vi "Create Unique Child Item Name.vi"(8 "error in (no error)":errorcluster, 10 "Name in":string, 11 "Parent Item Ref in":T1=18446744073709551615 format="%.0x") -> (0 "error out":errorcluster, 2 "Unique Name out":string, 3 "Parent Item Ref out":T1=18446744073709551615 format="%.0x")   [LabVIEW 2015, in "Waveform Data Logger System Explorer.lvlib"]
uses:
  Waveform Data Logger System Explorer.lvlib
  <vilib>/NI Veristand/Custom Device API/Custom Device Item Ref.ctl
  <vilib>/NI VeriStand/Custom Device API/Custom Device API.lvlib
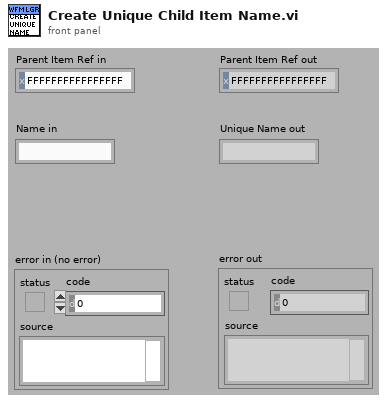
[diagram p1: front panel]
types:
  T1 = typedef "Custom Device API.lvlib/Custom Device Item Ref.ctl" = u64
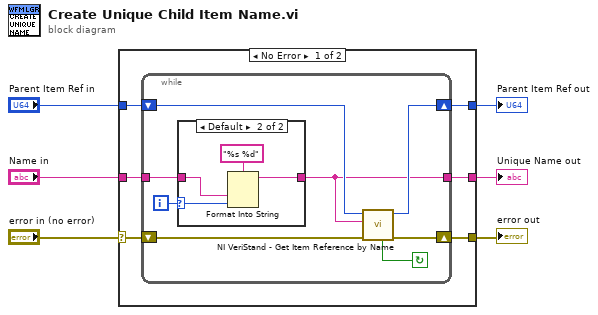
[diagram p0: block diagram]
diagram:
  n1 = case shown="No Error" "error in (no error)" {
    selector: "error in (no error)" -> [w12 w27]
    tunnel: [w11 w27] -> w5
    tunnel: "Parent Item Ref in" -> [w10 w26]
    tunnel: [w9 w26] -> w3
    tunnel: "Name in" -> [w8 _]
    tunnel: [w7 _] -> w1
    frame No Error {
      n2 = while {
        shift-right: [w14] -> w11
        shift-left: w12 -> [w18]
        shift-right: [w16] -> w9
        shift-left: w10 -> [w17]
        tunnel: w8 -> [w19]
        tunnel: [w13] -> w7
        i -> [w20]
        stop <- w15 continue-if-true
        n3 = case shown="Default" w20 {
          selector: w20 -> [_ w23]
          tunnel: w19 -> [w21 w24]
          tunnel: [w21 w22] -> w13
          frame 0 {
          }
          frame Default {
            n4 = Format Into String(format string="%s %d", w24, w23) -> (resulting string=w22:string)  [unwired: 2 in, 1 out]
          }
        }
        n5 = call <vilib>:"NI VeriStand - Get Item Reference by Name.vi"("error in (no error)"=w18, "Item Name"=w13, "Parent Ref in"=w17) -> ("error out"=w14:errorcluster, "Parent Ref out"=w16:T1, "Found"=w15:bool)  [unwired: 6 out]
      }
    }
    frame Error {
    }
  }
  "error out" <- w5
  "Unique Name out" <- w1
  "Parent Item Ref out" <- w3
